vi "Optitrack Position Client.vi"() -> (2 "Position XYZ":dbl[](array[numeric]) format="%.2f", 3 "Live?":bool, 4 "error out":errorcluster)   [LabVIEW 2021]
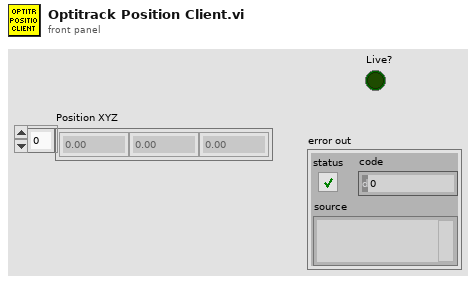
[diagram p1: front panel]
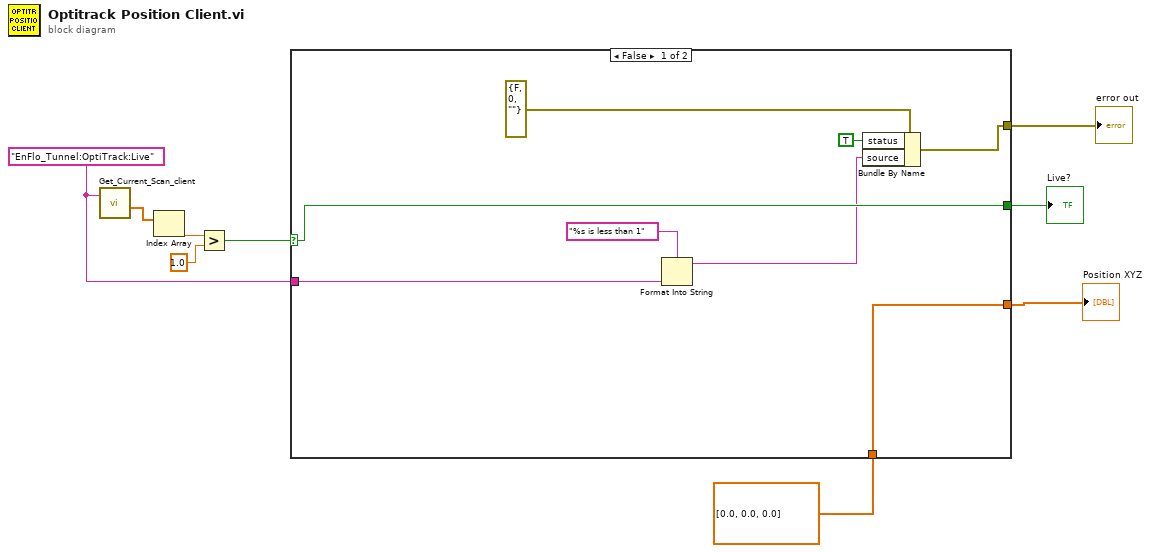
[diagram p0: block diagram]
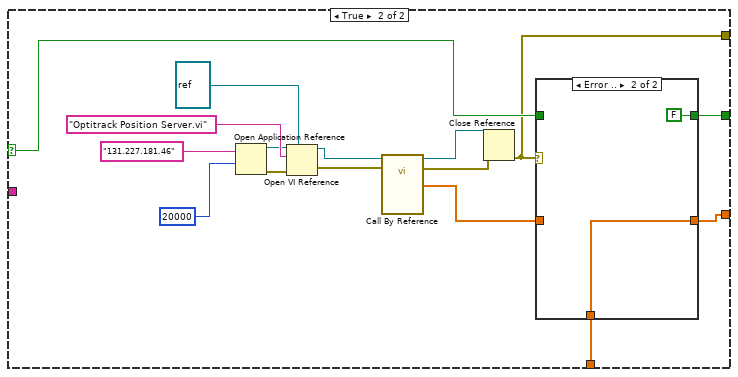
[diagram p2: hidden frame]
diagram:
  w1 = "EnFlo_Tunnel:OptiTrack:Live"
  n1 = call "Get_Current_Scan_client.vi"("singleChannel"=w1) -> ("Numerical Values"=w8:dbl[])  [unwired: 1 in, 3 out]
  n2 = Index Array(array=w8) -> (element=w7:dbl)  [unwired: 1 in]
  n3 = Greater?(x=w7, y=1.0) -> (0:w5:bool)
  n4 = case shown="False" w5 {
    selector: w5 -> [w16 w19]
    tunnel: [w17 w22] -> w9
    tunnel: dbl[] [0.0, 0.0, 0.0] ("Position XYZ") -> [w17 w21]
    tunnel: [w16 w20] -> w3
    tunnel: [w14 w18] -> w2
    tunnel: w1 -> [w12 _]
    frame False {
      n5 = Format Into String(format string="%s is less than 1", w12) -> (resulting string=w10:string)  [unwired: 2 in, 1 out]
      n6 = Bundle By Name(cluster=errorcluster {"status"=FALSE, "code"=0, "source"=""} ("error out"), "status"=TRUE, "source"=w10) -> (w14:errorcluster)
    }
    frame True {
      n7 = Open Application Reference(9:20000 ("timeout ms (60000)"), 11:"131.227.181.46" ("machine name (\"\":  open local reference)")) -> (0:w26:errorcluster, 3:w25:refnum<vi>)  [unwired: 2 in]
      n8 = Open VI Reference(type specifier VI Refnum (for type only)=refnum<vi> refnum ("Scout Server"), application reference (local)=w25, vi path="Optitrack Position Server.vi", error in (no error)=w26) -> (vi reference=w29:refnum<vi>, error out=w30:errorcluster)  [unwired: 2 out]
      n9 = call-by-ref "?"(reference=w29, error in=w30) -> (reference out=w31:refnum<vi>, error out=w32:errorcluster, "Position XYZ"=w23:dbl[])  [unwired: 3 in]
      n10 = Close Reference(reference=w31, error in (no error)=w32) -> (error out=w18:errorcluster)
      n11 = case shown="Error .." w18 {
        tunnel: w23 -> [w35 _]
        tunnel: [w35 w37] -> w22
        tunnel: w21 -> [_ w37]
        tunnel: [w34 FALSE] -> w20
        tunnel: w19 -> [w34 _]
        frame No Error {
        }
        frame Error {
        }
      }
    }
  }
  "Position XYZ" <- w9
  "Live?" <- w3
  "error out" <- w2
